vi "CreateMaze.vi"(8 "error in (no error)":errorcluster, 11 "MazeGame in":refnum<class "MazeGame.lvclass">) -> (0 "error out":errorcluster, 2 "Maze":refnum<class "Maze.lvclass">, 3 "MazeGame out":refnum<class "MazeGame.lvclass">)   [LabVIEW 2020, in "FactoryMethod.lvlib" / "NoParametrizedFactoryMethod.lvlib" / "MazeGame.lvclass"]
uses:
  MazeGame.lvclass
  GoFcommonClasses/Maze/Maze.lvclass
  GoFcommonClasses/Direction.ctl
  Private/TypeDef/RoomElement.ctl
  GoFcommonClasses/MazeSite/MazeSite.lvclass
  GoFcommonClasses/ConcreteMazeSite/Door/Door.lvclass
  E:/Francesco/GitHub/Design-Patterns-GoF_-_NI-LV/Creational/GoFcommonClasses/MazeSite/MazeSite.lvclass
  GoFcommonClasses/ConcreteMazeSite/Room/Room.lvclass
  Support/Class/ConsoleOutput.lvclass
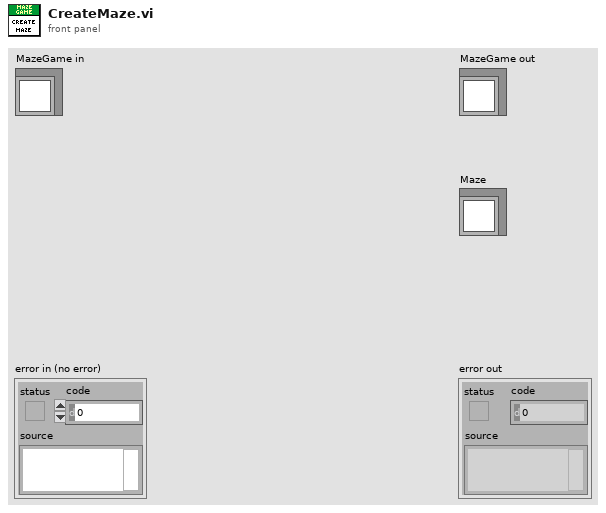
[diagram p1: front panel]
types:
  T1 = typedef "Room.lvclass/RoomElement.ctl" = cluster{"Direction":T2, "MazeSite":refnum<class "MazeSite.lvclass">}
  T2 = typedef "Direction.ctl" = enum32{"North", "South", "East", "West"}
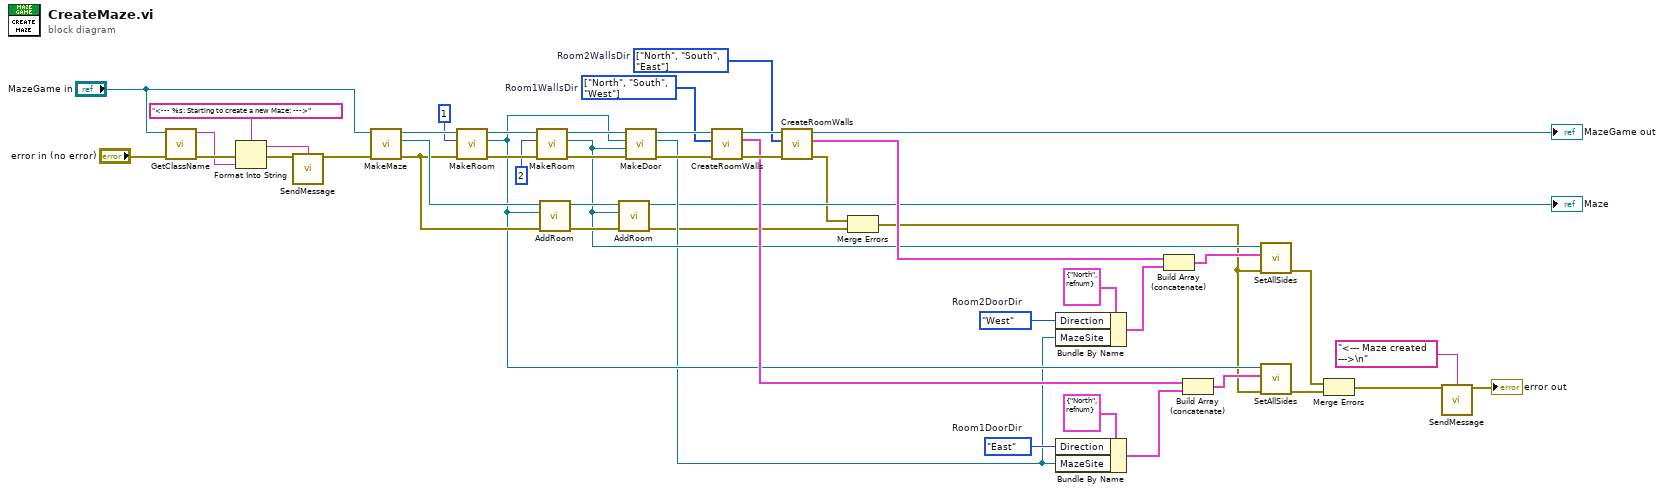
[diagram p0: block diagram]
diagram:
  w44 = Direction."West"  # Room2DoorDir
  w45 = Direction."East"  # Room1DoorDir
  w21 = T2[] [enum."North", enum."South", enum."East"] items=["North", "South", "East", "West"]  # Room2WallsDir
  w22 = T2[] [enum."North", enum."South", enum."West"] items=["North", "South", "East", "West"]  # Room1WallsDir
  n1 = call "GetClassName.vi"("error in (no error)"="error in (no error)", "object"="MazeGame in") -> ("error out"=w7:errorcluster, "Class Name"=w5:string)  [unwired: 8 in]
  n2 = Format Into String(format string="<--- %s: Starting to create a new Maze: --->" ("Message"), error in=w7, w5) -> (resulting string=w3:string, error out=w4:errorcluster)  [unwired: 1 in]
  n3 = call "SendMessage.vi"("Message"=w3, "error in (no error)"=w4) -> ("error out"=w26:errorcluster)  [unwired: 13 in]
  n4 = call-dynamic "MakeMaze.vi"("error in (no error)"=w26, "MazeGame in"="MazeGame in") -> ("error out"=w25:errorcluster, "Maze"=w27:refnum<class "Maze.lvclass">, "MazeGame out"=w33:refnum<class "MazeGame.lvclass">)  [unwired: 7 in]
  n5 = call-dynamic "MakeRoom.vi"("error in (no error)"=w25, "RoomNumber"=1, "MazeGame in"=w33) -> ("error out"=w34:errorcluster, "Room"=w17:refnum<class "Room.lvclass">, "MazeGame out"=w32:refnum<class "MazeGame.lvclass">)  [unwired: 6 in]
  n6 = call-dynamic "MakeRoom.vi"("error in (no error)"=w34, "RoomNumber"=2, "MazeGame in"=w32) -> ("error out"=w29:errorcluster, "Room"=w18:refnum<class "Room.lvclass">, "MazeGame out"=w28:refnum<class "MazeGame.lvclass">)  [unwired: 6 in]
  n7 = call "AddRoom.vi"("error in (no error)"=w25, "Room"=w17, "Maze in"=w27) -> ("error out"=w48:errorcluster, "Maze out"=w47:refnum<class "Maze.lvclass">)  [unwired: 7 in]
  n8 = call "AddRoom.vi"("error in (no error)"=w48, "Room"=w18, "Maze in"=w47) -> ("error out"=w14:errorcluster, "Maze out"=→"Maze":refnum<class "Maze.lvclass">)  [unwired: 7 in]
  n9 = call-dynamic "MakeDoor.vi"("error in (no error)"=w29, "Room 2"=w18, "Room 1"=w17, "MazeGame in"=w28) -> ("error out"=w24:errorcluster, "Door"=w16:refnum<class "Door.lvclass">, "MazeGame out"=w23:refnum<class "MazeGame.lvclass">)  [unwired: 5 in]
  n10 = call "CreateRoomWalls.vi"("error in (no error)"=w24, "DirectionsList"=w22, "MazeGame in"=w23) -> ("error out"=w38:errorcluster, "RoomWallsList"=w19:T1[], "MazeGame out"=w37:refnum<class "MazeGame.lvclass">)  [unwired: 6 in]
  n11 = call "CreateRoomWalls.vi"("error in (no error)"=w38, "DirectionsList"=w21, "MazeGame in"=w37) -> ("error out"=w13:errorcluster, "RoomWallsList"=w20:T1[], "MazeGame out"=→"MazeGame out":refnum<class "MazeGame.lvclass">)  [unwired: 6 in]
  n12 = Merge Errors(w13, w14) -> (w12:errorcluster)
  n13 = Bundle By Name(cluster=T1 {"Direction"=enum."North", "MazeSite"=refnum} ("RoomElement"), "Direction"=w44, "MazeSite"=w16) -> (w41:T1)
  n14 = Bundle By Name(cluster=T1 {"Direction"=enum."North", "MazeSite"=refnum} ("RoomElement"), "Direction"=w45, "MazeSite"=w16) -> (w42:T1)
  n15 = Build Array (concatenate)(w20, w41) -> (w36:T1[])
  n16 = Build Array (concatenate)(w19, w42) -> (w35:T1[])
  n17 = call "SetAllSides.vi"("error in (no error)"=w12, "RoomSides"=w36, "Room in"=w18) -> ("error out"=w40:errorcluster)  [unwired: 7 in, 1 out]
  n18 = call "SetAllSides.vi"("error in (no error)"=w12, "RoomSides"=w35, "Room in"=w17) -> ("error out"=w39:errorcluster)  [unwired: 7 in, 1 out]
  n19 = Merge Errors(w40, w39) -> (w2:errorcluster)
  n20 = call "SendMessage.vi"("Message"="<--- Maze created --->\n" ("format string"), "error in (no error)"=w2) -> ("error out"=→"error out":errorcluster)  [unwired: 13 in]
